vi "NormalBeam.vi"() -> ()   [LabVIEW 2017]
uses:
  <vilib>/Math Plots/2D Math Plots/XY Plot Matrix/XY Plot Matrix XCtrl/XY Plot Matrix.xctl
  <vilib>/ULx/Create Channel.llb/ULx Create Channel (AI-Voltage-Basic).vi
  <vilib>/ULx/Timing.llb/ULx Timing (Sample Clock).vi
  <vilib>/ULx/Read.llb/ULx Read (Analog Wfm 1Chan NSamp).vi
  <vilib>/Analysis/Matrix/Numeric/Conversions/Array To Matrix - RA.vi
  <vilib>/Math Plots/2D Math Plots/XY Plot Matrix/XY Plot Matrix Datatype/XY Plot Matrix Datatype.lvclass
  <vilib>/Analysis/Matrix/NI_Matrix.lvlib
panel:
  out "Stabalization Meter":dbl(knob) scale=-5.0..5.0
  out "Elements Cleared":i32
  in  "Clear Table":bool
  out "Weight To Be Added":dbl
  out "Weight Difference":dbl
  out "Weight Scale":dbl[](array[numeric])
  out "XY Plot Matrix":refnum<class "XY Plot Matrix Datatype.lvclass">[](xcontrol)
  out "Number of Sample":dbl format="%.0g"
  out "Voltage":dbl
  out "Voltage":dbl[](array[numeric])
  in  "Number of Calibrations":i8
  in  "Maximum Weight":dbl
  in  "Minimum Weight":dbl
  in  "Sample":bool
  in  "rate":dbl=1000.0
  in  "samples per channel":i32=1000
  in  "sample mode":i32(ring) items=["FiniteSamples", "ContinuousSamples"]
  in  "minimum value":dbl=-5.0
  in  "maximum value":dbl=5.0
  in  "physical channels":refnum<k21>
  # "Normal Beam"
  # "What is the range of your calibration?"
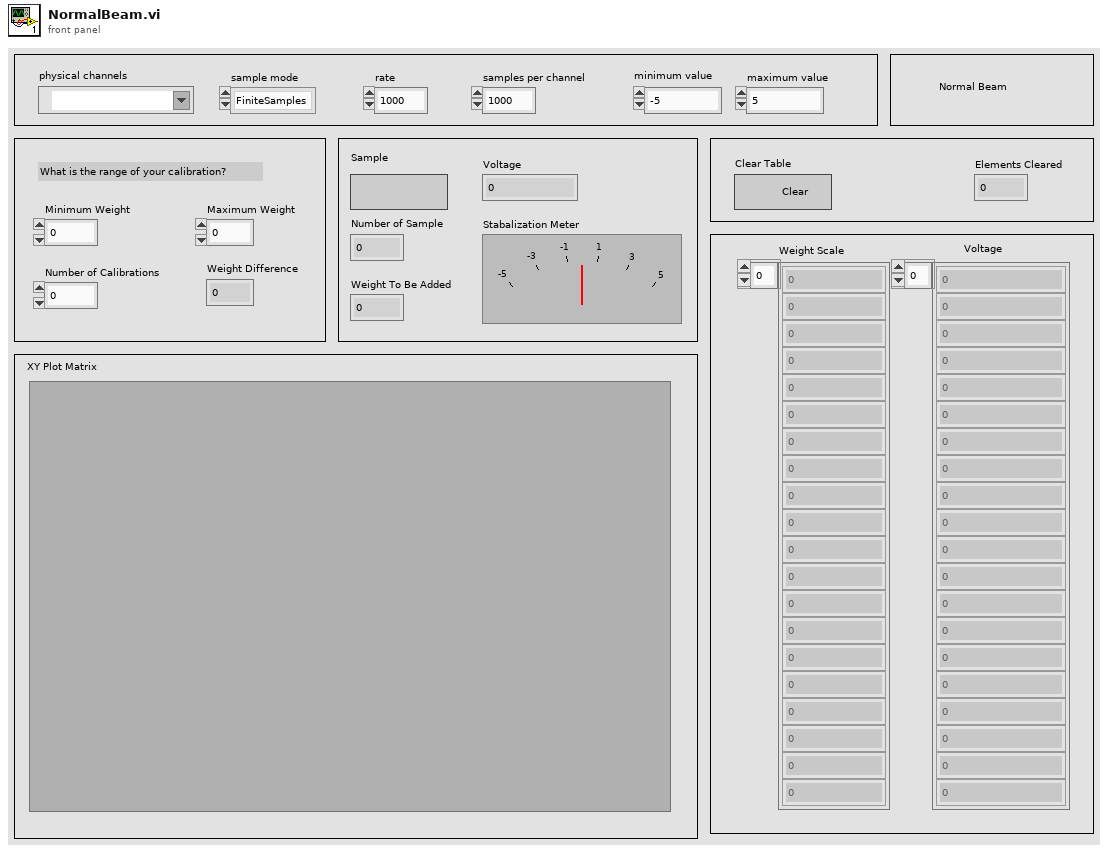
[diagram p1: front panel]
types:
  T1 = typedef "NI_Matrix.lvlib/RealMatrix.ctl" = dbl[][]
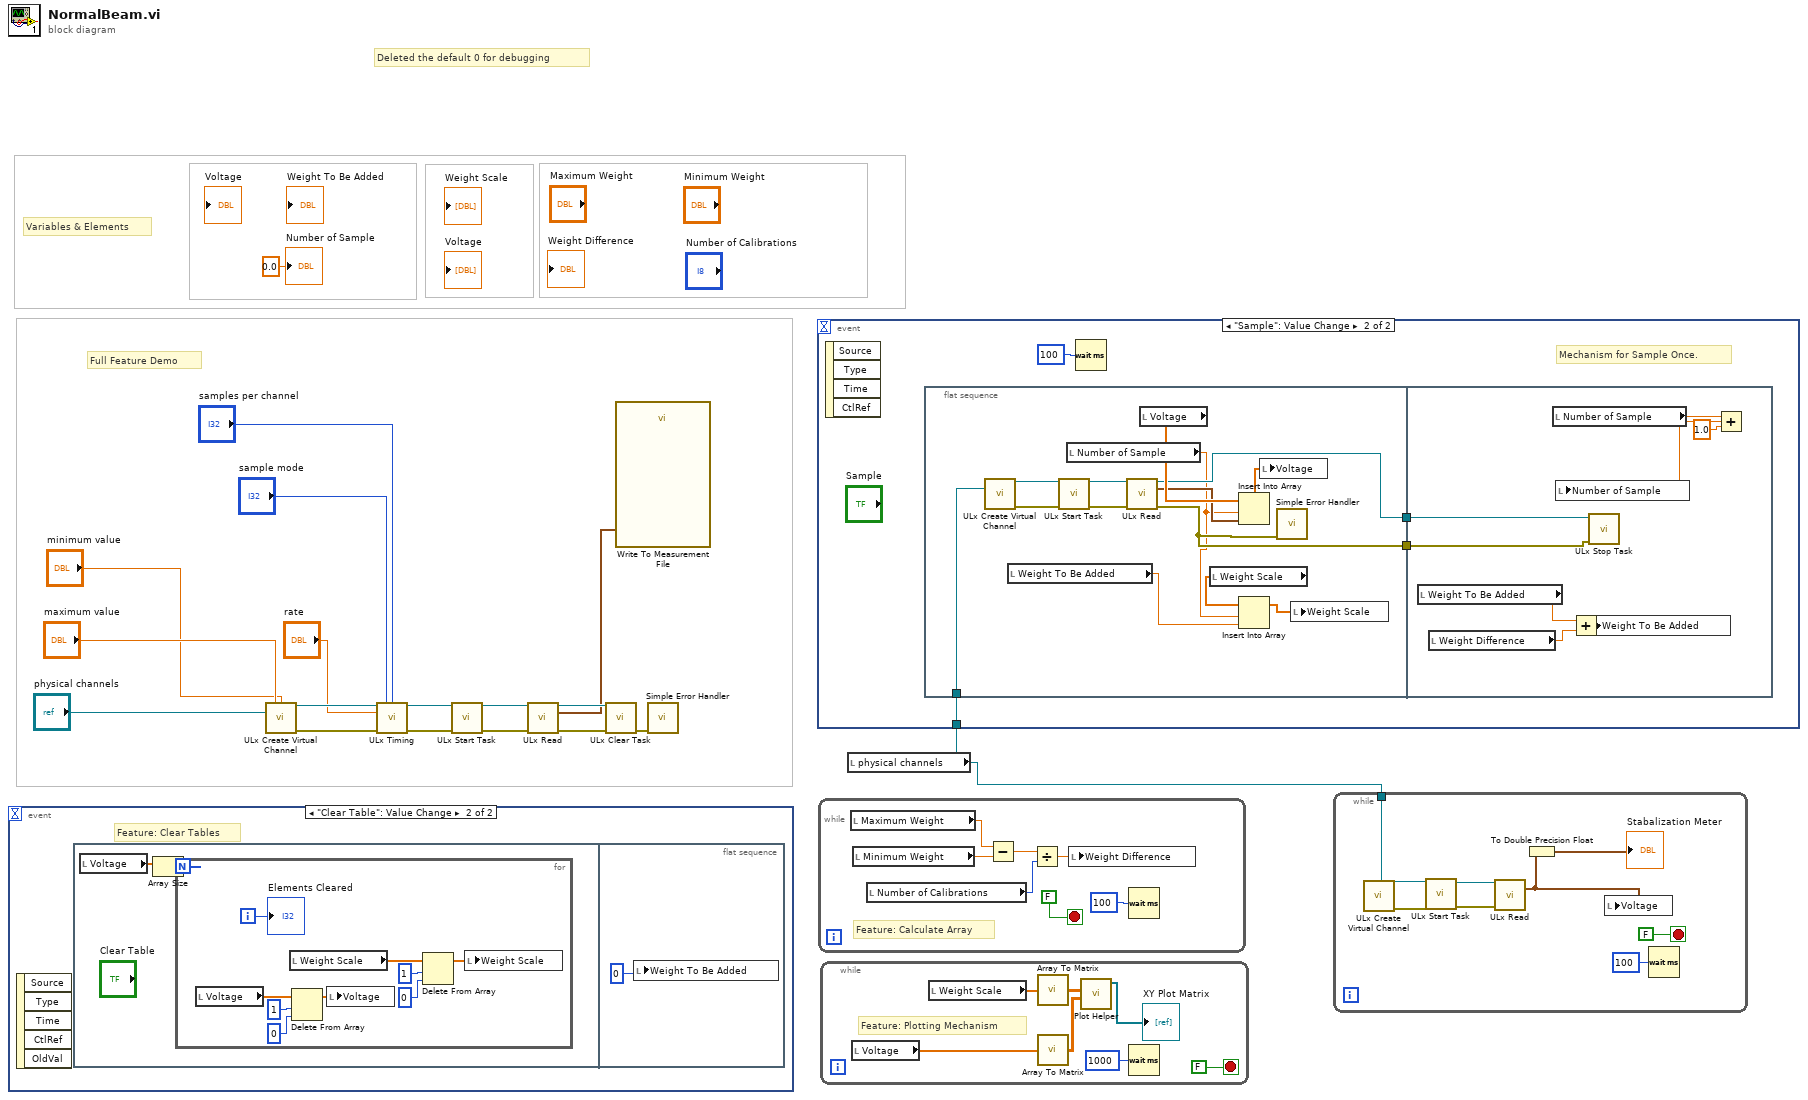
[diagram p0: block diagram]
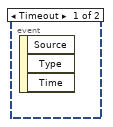
[diagram p2: hidden frame]
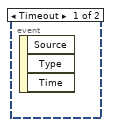
[diagram p3: hidden frame]
diagram:
  # "Deleted the default 0 for debugging"
  # "Full Feature Demo"
  # "Variables & Elements"
  n1 = event shown="[1] \"Clear Table\": Value Change" {
    selector: _ -> [_ _]
    dyn-events: _ -> [_ _]
    timeout: _ -> [_ _]
    event Timeout {
      n2 = event-data() -> ()  [unwired: 1 in, 3 out]
    }
    event "Clear Table": Value Change {
      # "Feature: Clear Tables"
      n3 = event-data() -> ()  [unwired: 1 in, 5 out]
      n4 = flat-sequence {
        frame #0 {
          n5 = local read "Voltage"() -> (w20:dbl[])
          n6 = Array Size(array=w20) -> (size(s)=w19:i32)
          n7 = for {
            N: w19 -> [_]
            i -> [w25]
            n8 = local read "Voltage"() -> (w29:dbl[])
            n9 = local read "Weight Scale"() -> (w27:dbl[])
            n10 = Delete From Array(array=w29, length=1, index=0) -> (array with subset deleted=w28:dbl[])  [unwired: 1 out]
            n11 = local write "Voltage"(w28) -> ()
            n12 = Delete From Array(array=w27, length=1, index=0) -> (array with subset deleted=w26:dbl[])  [unwired: 1 out]
            n13 = local write "Weight Scale"(w26) -> ()
            "Elements Cleared" <- w25
          }
        }
        frame #1 {
          n14 = local write "Weight To Be Added"(0) -> ()
        }
      }
    }
  }
  n15 = call-poly <vilib>:"ULx Create Virtual Channel.vi"("maximum value"="maximum value", "minimum value"="minimum value", "physical channels"="physical channels") -> ("task out"=w13:refnum<k24>, "error out"=w12:errorcluster)  [unwired: 11 in]
  n16 = call-poly <vilib>:"ULx Timing.vi"("task in"=w13, "sample mode"="sample mode", "samples per channel"="samples per channel", "rate"="rate", "error in"=w12) -> ("task out"=w10:refnum<k24>, "error out"=w9:errorcluster)  [unwired: 9 in]
  n17 = call <vilib>:"ULx Start Task.vi"("task in"=w10, "error in"=w9) -> ("task out"=w8:refnum<k24>, "error out"=w7:errorcluster)  [unwired: 12 in]
  n18 = call-poly <vilib>:"ULx Read.vi"("task in"=w8, "error in"=w7) -> ("task out"=w6:refnum<k24>, "data"=w3:waveform(dbl), "error out"=w5:errorcluster)  [unwired: 11 in]
  n19 = call <vilib>:"ULx Clear Task.vi"("task in"=w6, "error in"=w5) -> ("error out"=w4:errorcluster)  [unwired: 13 in]
  n20 = call "Write To Measurement File"("Signals"=w3) -> ()  [unwired: 16 in, 3 out]
  n21 = call <vilib>:"Simple Error Handler.vi"("error in (no error)"=w4) -> ()  [unwired: 4 in, 5 out]
  n22 = while {
    stop <- FALSE stop-if-true
    # "Feature: Calculate Array"
    n23 = local read "Maximum Weight"() -> (w35:dbl)
    n24 = local read "Minimum Weight"() -> (w34:dbl)
    n25 = local read "Number of Calibrations"() -> (w32:i8)
    n26 = Subtract(x=w35, y=w34) -> (x-y=w33:dbl)
    n27 = Divide(x=w33, y=w32) -> (x/y=w31:dbl)
    n28 = local write "Weight Difference"(w31) -> ()
    n29 = Wait (ms)(milliseconds to wait=u32 100) -> ()  [unwired: 1 out]
  }
  n30 = while {
    stop <- FALSE stop-if-true
    # "Feature: Plotting Mechanism"
    n31 = local read "Voltage"() -> (w41:dbl[])
    n32 = local read "Weight Scale"() -> (w42:dbl[])
    n33 = call-poly <vilib>:"Array To Matrix.vi"("Real 1D Array"=w42) -> ("Real Matrix (Column Vector)"=w44:T1)
    n34 = call-poly <vilib>:"Array To Matrix.vi"("Real 1D Array"=w41) -> ("Real Matrix (Column Vector)"=w43:T1)
    n35 = call <vilib>:"Plot Helper.vi"("y matrix"=w43, "x matrix"=w44) -> ("2D Plotmatrix Class Obj Array out"=→"XY Plot Matrix":refnum<class "XY Plot Matrix Datatype.lvclass">[])  [unwired: 2 in, 7 out]
    n36 = Wait (ms)(milliseconds to wait=u32 1000) -> ()  [unwired: 1 out]
  }
  n37 = local read "physical channels"() -> (w1:refnum<k21>)
  n38 = event shown="[1] \"Sample\": Value Change" {
    selector: _ -> [_ _]
    dyn-events: _ -> [_ _]
    timeout: _ -> [_ _]
    tunnel: w1 -> [_ w45]
    event Timeout {
      n39 = event-data() -> ()  [unwired: 1 in, 3 out]
    }
    event "Sample": Value Change {
      # "Mechanism for Sample Once."
      n40 = event-data() -> ()  [unwired: 1 in, 4 out]
      n41 = flat-sequence {
        tunnel: [w55] -> w47
        tunnel: [w54] -> w46
        tunnel: w45 -> [w49]
        tunnel: w47 -> [w67]
        tunnel: w46 -> [w66]
        frame #0 {
          n42 = call-poly <vilib>:"ULx Create Virtual Channel.vi"("physical channels"=w49) -> ("task out"=w60:refnum<k24>, "error out"=w57:errorcluster)  [unwired: 13 in]
          n43 = local read "Weight To Be Added"() -> (w50:dbl)
          n44 = call <vilib>:"ULx Start Task.vi"("task in"=w60, "error in"=w57) -> ("task out"=w59:refnum<k24>, "error out"=w58:errorcluster)  [unwired: 12 in]
          n45 = local read "Number of Sample"() -> (w52:dbl)
          n46 = call-poly <vilib>:"ULx Read.vi"("task in"=w59, "error in"=w58) -> ("task out"=w54:refnum<k24>, "data"=w56:waveform(dbl), "error out"=w55:errorcluster)  [unwired: 11 in]
          n47 = local read "Voltage"() -> (w61:dbl[])
          n48 = local read "Weight Scale"() -> (w53:dbl[])
          n49 = Insert Into Array(array=w61, index=w52, new element=w56) -> (w62:dbl[])
          n50 = Insert Into Array(array=w53, index=w52, new element=w50) -> (w51:dbl[])
          n51 = local write "Voltage"(w62) -> ()
          n52 = call <vilib>:"Simple Error Handler.vi"("error in (no error)"=w55) -> ()  [unwired: 4 in, 5 out]
          n53 = local write "Weight Scale"(w51) -> ()
        }
        frame #1 {
          n54 = local read "Weight To Be Added"() -> (w65:dbl)
          n55 = local read "Weight Difference"() -> (w64:dbl)
          n56 = local read "Number of Sample"() -> (w70:dbl)
          n57 = Add(x=w65, y=w64) -> (x+y=w63:dbl)
          n58 = local write "Weight To Be Added"(w63) -> ()
          n59 = call <vilib>:"ULx Stop Task.vi"("error in"=w67, "task in"=w66) -> ()  [unwired: 8 in, 2 out]
          n60 = Add(x=w70, y=1.0) -> (x+y=w69:dbl)
          n61 = local write "Number of Sample"(w69) -> ()
        }
      }
      n62 = Wait (ms)(milliseconds to wait=u32 100) -> ()  [unwired: 1 out]
    }
  }
  n63 = while {
    tunnel: w1 -> [w73]
    stop <- FALSE stop-if-true
    n64 = call-poly <vilib>:"ULx Create Virtual Channel.vi"("physical channels"=w73) -> ("task out"=w79:refnum<k24>, "error out"=w78:errorcluster)  [unwired: 13 in]
    n65 = call <vilib>:"ULx Start Task.vi"("task in"=w79, "error in"=w78) -> ("task out"=w77:refnum<k24>, "error out"=w76:errorcluster)  [unwired: 12 in]
    n66 = call-poly <vilib>:"ULx Read.vi"("task in"=w77, "error in"=w76) -> ("data"=w72:waveform(dbl))  [unwired: 11 in, 2 out]
    n67 = To Double Precision Float(number=w72) -> (double precision float=→"Stabalization Meter":waveform(dbl))
    n68 = local write "Voltage"(w72) -> ()
    n69 = Wait (ms)(milliseconds to wait=u32 100) -> ()  [unwired: 1 out]
  }
  "Number of Sample" <- 0.0 ("Number of Sample")
